vi "Write Counting Gates.vi"(10 "Counting Gates":T1, 11 "User Interface in":refnum<class "User Interface.lvclass">) -> (3 "User Interface out":refnum<class "User Interface.lvclass">)   [LabVIEW 2016, in "_User Interface.lvlib" / "User Interface.lvclass"]
uses:
  User Interface.lvclass
  Counter Parameters.ctl
  _User Interface.lvlib
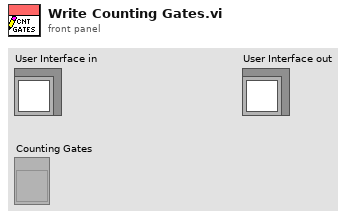
[diagram p1: front panel]
types:
  T1 = typedef "_User Interface.lvlib/Counter Parameters.ctl" = refnum<vi>
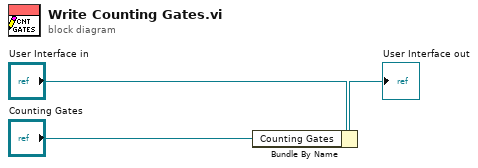
[diagram p0: block diagram]
diagram:
  n1 = Bundle By Name(cluster="User Interface in", "Counting Gates"="Counting Gates") -> (→"User Interface out":refnum<class "User Interface.lvclass">)
